vi "CHR17040 Battery Pack.vi"   [LabVIEW 2018]
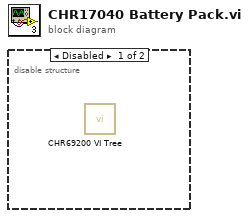
[diagram p0: block diagram]
diagram:
  n1 = disable-structure shown="Disabled" {
    frame Disabled {
      n2 = call <instrlib>:"CHR69200 VI Tree.vi"() -> ()  [unwired: 12 in]
    }
    frame Enabled {
    }
  }
